vi "主UI.vi"() -> ()   [LabVIEW 2016, in "自动更新.lvlib" / "TCP文件传输系统.lvlib"]
uses:
  <vilib>/Utility/sysdir.llb/System Directory Type.ctl
panel:
  out "TCP接收全局簇":T1
  out "TCP发送全局簇":T2
  out "传输次数":dbl
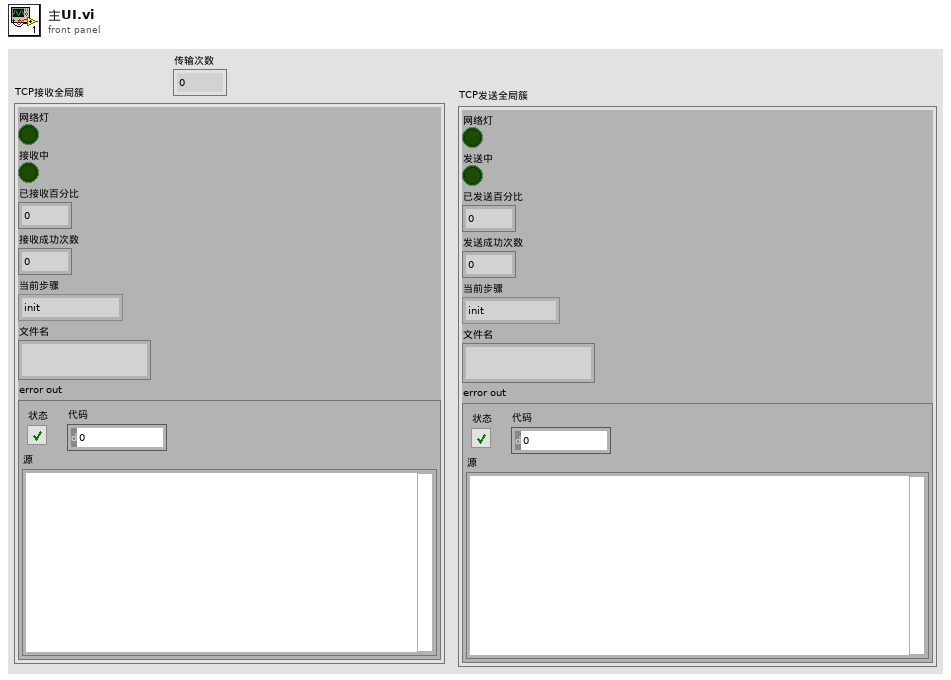
[diagram p1: front panel]
types:
  T1 = cluster{"网络灯":bool, "接收中":bool, "已接收百分比":u8, "接收成功次数":dbl, "当前步骤":enum16{"init", "receivehead", "receivecontent", "receivesuccess", "over"}, "文件名":string, "error out":errorcluster}
  T2 = cluster{"网络灯":bool, "发送中":bool, "已发送百分比":u8, "发送成功次数":dbl, "当前步骤":enum16{"init", "sendhead", "sendcontent", "sendsuccess", "over"}, "文件名":string, "error out":errorcluster}
  T3 = typedef "System Directory Type.ctl" = i32
  T4 = cluster{"网络灯":bool, "发送中":bool, "已发送百分比":u8, "发送成功次数":dbl, "当前步骤":enum16{"readfile", "init", "sendhead", "sendcontent", "sendsuccess", "over"}, "文件名":string, "error out":errorcluster}
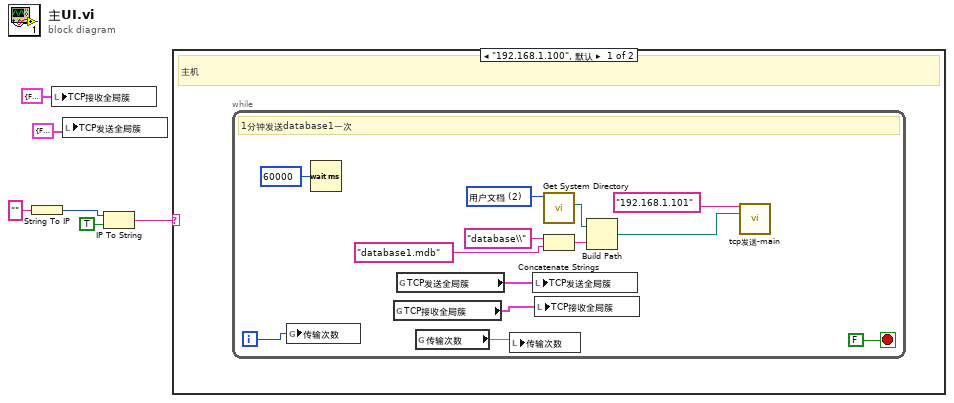
[diagram p0: block diagram]
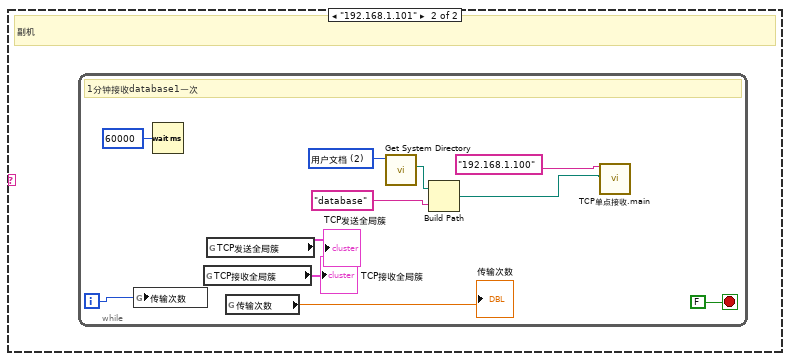
[diagram p2: hidden frame]
diagram:
  n1 = String To IP(1:"" ("名称")) -> (0:w6:u32)
  n2 = local write "TCP接收全局簇"(T1 {"网络灯"=FALSE, "接收中"=FALSE, "已接收百分比"=0, "接收成功次数"=0.0, "当前步骤"=enum."init", "文件名"="", "error out"={"status"=FALSE, "code"=0, "source"=""}} ("TCP接收全局簇")) -> ()
  n3 = local write "TCP发送全局簇"(T2 {"网络灯"=FALSE, "发送中"=FALSE, "已发送百分比"=0, "发送成功次数"=0.0, "当前步骤"=enum."init", "文件名"="", "error out"={"status"=FALSE, "code"=0, "source"=""}} ("TCP发送全局簇")) -> ()
  n4 = IP To String(1:TRUE ("句点符号？(F)"), 2:w6) -> (0:w3:string)
  n5 = case shown="\"192.168.1.100\", 默认" w3 {
    frame "192.168.1.100", Default {
      # "主机"
      n6 = while {
        i -> [w10]
        stop <- FALSE stop-if-true
        w16 = T3 2 items=["用户目录"=0, "用户桌面"=1, "用户文档"=2, "用户应用程序数据"=3, "用户设置"=4, "用户临时目录"=5, "公共文档"=6, "公共应用程序数据"=7, "公共设置"=8, "公共缓存"=13, "系统核心库"=9, "系统安装库"=10, "应用程序文件"=11, "启动盘根目录"=12] ("system directory type")
        # "1分钟发送database1一次"
        n7 = global write "全局变量1.vi" "传输次数"(w10) -> ()
        n8 = Wait (ms)(milliseconds to wait=u32 60000 ("等待时间（毫秒）")) -> ()  [unwired: 1 out]
        n9 = global read "全局变量1.vi" "TCP接收全局簇"() -> (w7:T1)
        n10 = global read "全局变量1.vi" "TCP发送全局簇"() -> (w8:T4)
        n11 = global read "全局变量1.vi" "传输次数"() -> (w9:dbl)
        n12 = local write "传输次数"(w9) -> ()
        n13 = local write "TCP发送全局簇"(w8) -> ()
        n14 = local write "TCP接收全局簇"(w7) -> ()
        n15 = call <vilib>:"Get System Directory.vi"("system directory type"=w16) -> ("system directory"=w15:path)  [unwired: 10 in]
        n16 = Concatenate Strings("database\\" ("condition"), "database1.mdb" ("字符串")) -> (w13:string)
        n17 = Build Path(base path=w15, name or relative path=w13) -> (appended path=w11:path)
        n18 = call "tcp发送-main.vi"("服务器网络地址"="192.168.1.101" ("对方网络地址"), "原文件路径（使用对话框）"=w11) -> ()  [unwired: 12 in, 2 out]
      }
    }
    frame "192.168.1.101" {
      # "副机"
      n19 = while {
        i -> [w24]
        stop <- FALSE stop-if-true
        w28 = T3 2 items=["用户目录"=0, "用户桌面"=1, "用户文档"=2, "用户应用程序数据"=3, "用户设置"=4, "用户临时目录"=5, "公共文档"=6, "公共应用程序数据"=7, "公共设置"=8, "公共缓存"=13, "系统核心库"=9, "系统安装库"=10, "应用程序文件"=11, "启动盘根目录"=12] ("system directory type")
        # "1分钟接收database1一次"
        n20 = global write "全局变量1.vi" "传输次数"(w24) -> ()
        n21 = Wait (ms)(milliseconds to wait=u32 60000 ("等待时间（毫秒）")) -> ()  [unwired: 1 out]
        n22 = global read "全局变量1.vi" "TCP接收全局簇"() -> (→"TCP接收全局簇":T1)
        n23 = global read "全局变量1.vi" "TCP发送全局簇"() -> (→"TCP发送全局簇":T4)
        n24 = global read "全局变量1.vi" "传输次数"() -> (→"传输次数":dbl)
        n25 = call <vilib>:"Get System Directory.vi"("system directory type"=w28) -> ("system directory"=w27:path)  [unwired: 10 in]
        n26 = Build Path(base path=w27, name or relative path="database" ("condition")) -> (appended path=w25:path)
        n27 = call "TCP单点接收.main.vi"("IP地址"="192.168.1.100" ("对方网络地址"), "储存路径"=w25) -> ()  [unwired: 15 in, 3 out]
      }
    }
  }
